vi "Read AI DAQ Data.vi"(0 "DAQ Node Dict DVR":T3, 1 "AI TaskName":string, 2 "Public P&ID Events":T2, 3 "MainProc_ScanDataQ":T1, 5 "DAQ Data Dict DVR":T3, 7 "AI IONames":string[](array[string]), 9 "RawAIDataQ":T4, 11 "error in":errorcluster, 12 "Logger_ScanDataQ":T1) -> (4 "DAQ Node Dict DVR out":T3, 6 "DAQ Data Dict DVR out":T3, 15 "error out":errorcluster)   [LabVIEW 2017, in "DAQ.lvclass"]
doc: "Developed by Kevin Thompson\nkevin@thompsonengineering.net\n\nCopyright 2018-2020\nThompson Engineering, LLC\nAI scan timestamp is stored with IOName \"AIScanTS\" in DAQ Data Dict.\nAI scan array is stored with IOName \"AIScanArray\" in DAQ Data Dict.\n[AI IONames] input is obtained from AI IOName enum TD"
uses:
  DAQ.lvclass
  Support/DataQueues/DataTypes/Analog DataSet MultiRow--QRef.ctl
  Support/DataQueues/DataTypes/Analog DataSet MultiRow--cluster.ctl
  <vilib>/TELLC/Dynamic CVT API/TD Dynamic CVT DVR--ref.ctl
  Support/DataQueues/DataTypes/Analog DataSet MultiRow & ChanNames--QRef.ctl
  Support/DataQueues/DataTypes/Analog DataSet MultiRow & ChanNames--cluster.ctl
  Support/DataQueues/DataQueues.lvclass
panel:
  # "#NOTE: presently not used"
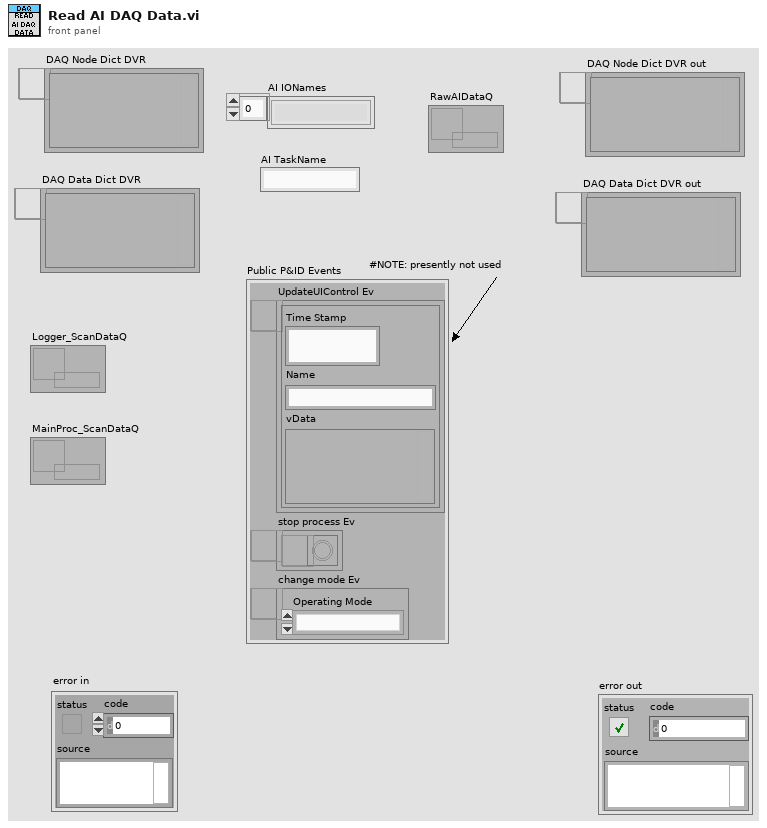
[diagram p1: front panel]
types:
  T1 = typedef "DataQueues.lvclass/Analog DataSet MultiRow & ChanNames--QRef.ctl" = refnum<queue>
  T2 = cluster{"UpdateUIControl Ev":refnum<user-event>, "stop process Ev":refnum<user-event>, "change mode Ev":refnum<user-event>}
  T3 = typedef "TD Dynamic CVT DVR--ref.ctl" = refnum<data-value>
  T4 = typedef "DataQueues.lvclass/Analog DataSet MultiRow--QRef.ctl" = refnum<queue>
  T5 = typedef "DataQueues.lvclass/Analog DataSet MultiRow & ChanNames--cluster.ctl" = cluster{"TimeStamp_(s)":dbl, "data":dbl[][], "ChanNames":string[]}
  T6 = typedef "DAQ.lvclass/TD local raw AI Data--cluster.ctl" = cluster{"TimeStamp_(s)":dbl, "data":dbl[][]}
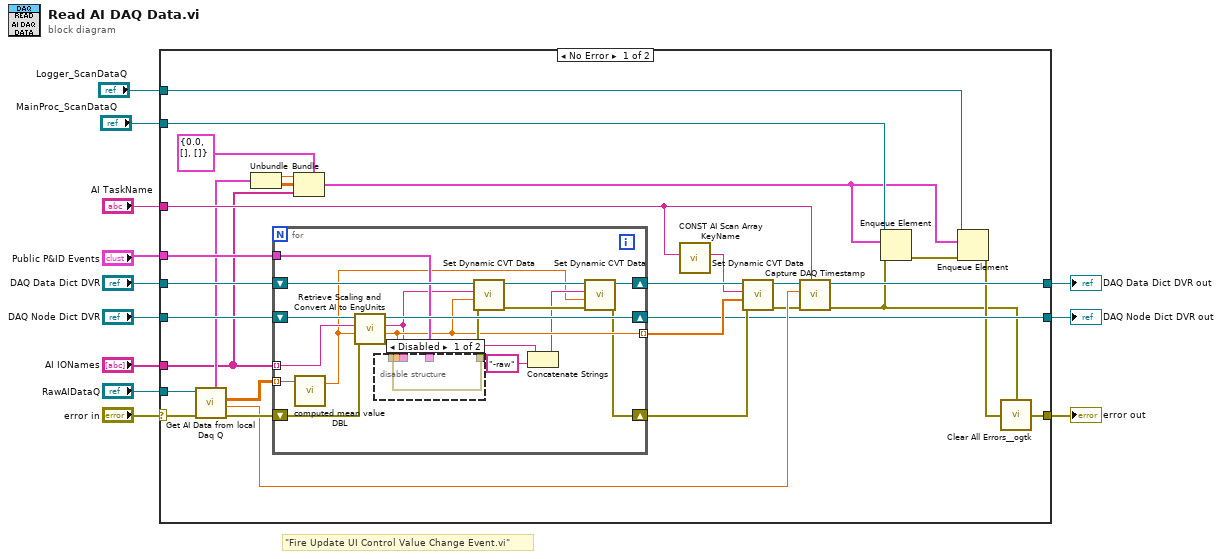
[diagram p0: block diagram]
diagram:
  # "\"Fire Update UI Control Value Change Event.vi\""
  n1 = case shown="No Error" "error in" {
    selector: "error in" -> [w36 w65]
    tunnel: "RawAIDataQ" -> [w37 _]
    tunnel: "DAQ Data Dict DVR" -> [w41 w66]
    tunnel: [w30 w66] -> w10
    tunnel: [w20 w65] -> w9
    tunnel: "DAQ Node Dict DVR" -> [w40 w64]
    tunnel: [w26 w64] -> w6
    tunnel: "AI IONames" -> [w15 _]
    tunnel: "AI TaskName" -> [w21 _]
    tunnel: "Public P&ID Events" -> [w29 _]
    tunnel: "MainProc_ScanDataQ" -> [w27 _]
    tunnel: "Logger_ScanDataQ" -> [w22 _]
    frame No Error {
      n2 = call "Get AI Data from local Daq Q.vi"("error in"=w36, "daqThread AI local Q"=w37) -> ("error out"=w39:errorcluster, "timestamp"=w38:dbl, "data"=w25:dbl[][], "Q element"=w18:T6)  [unwired: 5 in, 1 out]
      n3 = Unbundle(w18) -> ("TimeStamp_(s)"=w17:dbl, "data"=w16:dbl[][])
      n4 = for {
        tunnel: w25 -> [w59] mode=indexing
        tunnel: w15 -> [w54] mode=indexing
        shift-right: [w48] -> w35
        shift-left: w41 -> [w58]
        shift-right: [w46] -> w32
        shift-left: w39 -> [w56]
        shift-right: [w55] -> w26
        shift-left: w40 -> [w57]
        tunnel: [w50] -> w33 mode=indexing
        tunnel: w29 -> [w51]
        n5 = call <vilib>:"computed mean value DBL.vi"("Array in"=w59) -> ("MeanValue"=w42:dbl)  [unwired: 1 out]
        n6 = call "Retrieve Scaling and Convert AI to EngUnits.vi"("error in (no error)"=w56, "RawValue in"=w42, "IOName"=w54, "DAQ Node Dict DVR"=w57) -> ("error out"=w53:errorcluster, "Engineering Units Out"=w50:dbl, "IOName out"=w45:string, "DAQ Node Dict DVR out"=w55:T3)  [unwired: 4 in]
        n7 = disable-structure shown="Disabled" {
          disable-tunnel: w53 -> [w60 w63]
          disable-tunnel: [w60 w63] -> w52
          disable-tunnel: w51 -> [_ _]
          disable-tunnel: w50 -> [w62 _]
          disable-tunnel: w45 -> [w61 _]
          frame Disabled {
          }
          frame Enabled {
          }
        }
        n8 = call <vilib>:"Set Dynamic CVT Data.vi"("error in (no error)"=w52, "value"=w50, "DataName"=w45, "dCVT DVR"=w58) -> ("error out"=w47:errorcluster, "dCVT DVR out"=w49:T3)  [unwired: 5 in, 1 out]
        n9 = Concatenate Strings(w45, "-raw" ("string")) -> (w43:string)
        n10 = call <vilib>:"Set Dynamic CVT Data.vi"("error in (no error)"=w47, "value"=w42, "DataName"=w43, "dCVT DVR"=w49) -> ("error out"=w46:errorcluster, "dCVT DVR out"=w48:T3)  [unwired: 5 in, 1 out]
      }
      n11 = Bundle(cluster=T5 {"TimeStamp_(s)"=0.0, "data"=[], "ChanNames"=[]} ("Analog DataSet MultiRow & ChanNames"), "TimeStamp_(s)"=w17, "data"=w16, "ChanNames"=w15) -> (w14:T5)
      n12 = call "CONST AI Scan Array KeyName.vi"("AI TaskName"=w21) -> ("AI ScanArray (KeyName)"=w28:string)  [unwired: 10 in]
      n13 = call <vilib>:"Set Dynamic CVT Data.vi"("error in (no error)"=w32, "value"=w33, "DataName"=w28, "dCVT DVR"=w35) -> ("error out"=w31:errorcluster, "dCVT DVR out"=w34:T3)  [unwired: 5 in, 1 out]
      n14 = call "Capture DAQ Timestamp.vi"("DaqData dCVT"=w34, "timestamp in"=w38, "error in (no error)"=w31, "AI TaskName"=w21) -> ("DaqData dCVT out"=w30:T3, "error out"=w19:errorcluster)  [unwired: 4 in, 1 out]
      n15 = Enqueue Element(queue=w27, element=w14, error in (no error)=w19) -> (error out=w24:errorcluster)  [unwired: 1 in, 2 out]
      n16 = Enqueue Element(queue=w22, element=w14, error in (no error)=w24) -> (error out=w23:errorcluster)  [unwired: 1 in, 2 out]
      n17 = call <userlib>:"Clear All Errors__ogtk.vi"("Upsteam Error (optional)"=w19, "Error In"=w23) -> ("Error Out"=w20:errorcluster)  [unwired: 2 in]
    }
    frame Error {
    }
  }
  "DAQ Data Dict DVR out" <- w10
  "error out" <- w9
  "DAQ Node Dict DVR out" <- w6
